vi "Resource to String.vi"(8 "error in (no error)":errorcluster, 10 "Resource as Variant":variant, 11 "Generic Controller in":refnum<class "Generic Plugin.lvclass">) -> (0 "error out":errorcluster, 2 "Resource as String":string, 3 "Generic Controller out":refnum<class "Generic Plugin.lvclass">)   [LabVIEW 2020, in "RxnRover.lvlib" / "Generic Plugin.lvclass"]
uses:
  Generic Plugin.lvclass
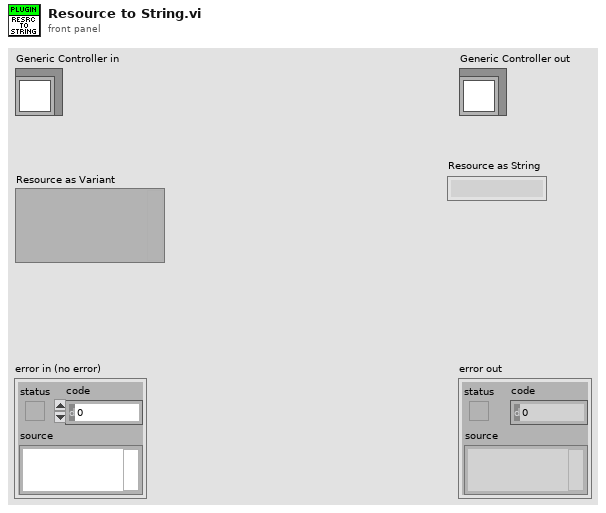
[diagram p1: front panel]
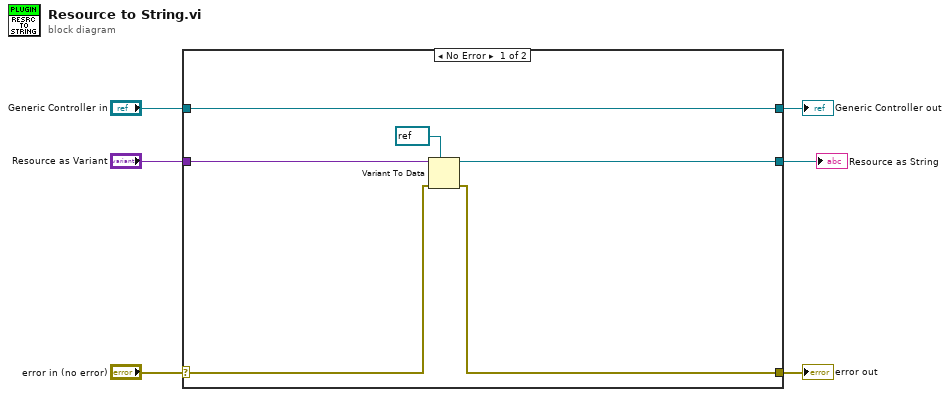
[diagram p0: block diagram]
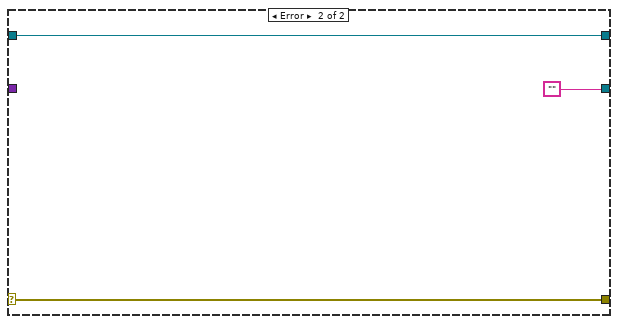
[diagram p2: hidden frame]
diagram:
  n1 = case shown="No Error" "error in (no error)" {
    selector: "error in (no error)" -> [w11 w15]
    tunnel: [w10 w15] -> w5
    tunnel: [w12 w14] -> w3
    tunnel: "Generic Controller in" -> [w12 w14]
    tunnel: "Resource as Variant" -> [w9 _]
    tunnel: [w8 ""] -> w1
    frame No Error {
      n2 = Variant To Data(error in=w11, type=refnum<visa-resource-name> refnum ("VISA resource name"), Variant=w9) -> (data=w8:refnum<visa-resource-name>, error out=w10:errorcluster)
    }
    frame Error {
    }
  }
  "error out" <- w5
  "Generic Controller out" <- w3
  "Resource as String" <- w1
